vi "ni579x Configure Amplifier.vi"(0 "Register Bus":refnum<class "ni579x Register Bus v1 Host.lvclass">=refnum, 1 "scope":string(combo)="rx", 5 "enable?":bool=TRUE, 11 "Error In":errorcluster) -> (4 "Register Bus (out)":refnum<class "ni579x Register Bus v1 Host.lvclass">, 6 "coerced enable":bool, 15 "Error Out":errorcluster)   [LabVIEW 2015]
uses:
  <instrlib>/ni579x/Register Bus/v1/Host/ni579x Register Bus v1 Host.lvclass
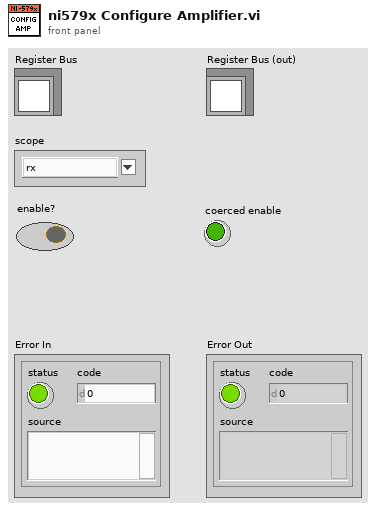
[diagram p1: front panel]
types:
  T1 = typedef "ni579x User Command.ctl" = cluster{"User Data 0":u8, "User Data 1":u8, "User Command ID":T2}
  T2 = typedef "ni579x User Command ID.ctl" = u8
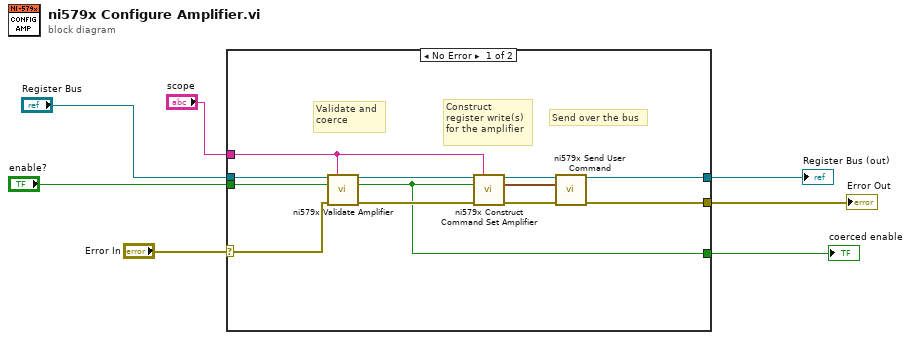
[diagram p0: block diagram]
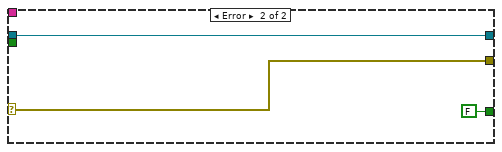
[diagram p2: hidden frame]
diagram:
  n1 = case shown="No Error" "Error In" {
    selector: "Error In" -> [w18 w22]
    tunnel: [w16 w22] -> w6
    tunnel: "Register Bus" -> [w19 w21]
    tunnel: "enable?" -> [w9 _]
    tunnel: [w17 w21] -> w4
    tunnel: "scope" -> [w12 _]
    tunnel: [w8 FALSE ("coerced enable")] -> w1
    frame No Error {
      # "Construct\nregister write(s)\nfor the amplifier"
      # "Send over the bus"
      # "Validate and \ncoerce"
      n2 = call <instrlib>:"ni579x Validate Amplifier.vi"("Register Bus"=w19, "scope"=w12, "enable?"=w9, "Error In"=w18) -> ("Register Bus (out)"=w11:refnum<class "ni579x Register Bus v1 Host.lvclass">, "coerced enable"=w8:bool, "Error Out"=w10:errorcluster)  [unwired: 9 in]
      n3 = call <instrlib>:"ni579x Construct Command Set Amplifier.vi"("Register Bus"=w11, "scope"=w12, "enabled?"=w8, "Error In"=w10) -> ("Register Bus (out)"=w15:refnum<class "ni579x Register Bus v1 Host.lvclass">, "User Command"=w14:T1, "Error Out"=w13:errorcluster)  [unwired: 9 in]
      n4 = call <instrlib>:"ni579x Send User Command.vi"("Register Bus"=w15, "User Command"=w14, "Error In"=w13) -> ("Register Bus (out)"=w17:refnum<class "ni579x Register Bus v1 Host.lvclass">, "Error Out"=w16:errorcluster)  [unwired: 8 in, 3 out]
    }
    frame Error {
    }
  }
  "Register Bus (out)" <- w4
  "Error Out" <- w6
  "coerced enable" <- w1
